vi "recycle_put.vi"(8 "Error In":errorcluster, 9 "Position In":T1) -> (0 "Error Out":errorcluster, 1 "Position out":T1)   [LabVIEW 2019]
uses:
  subVI/move/position cluster.ctl
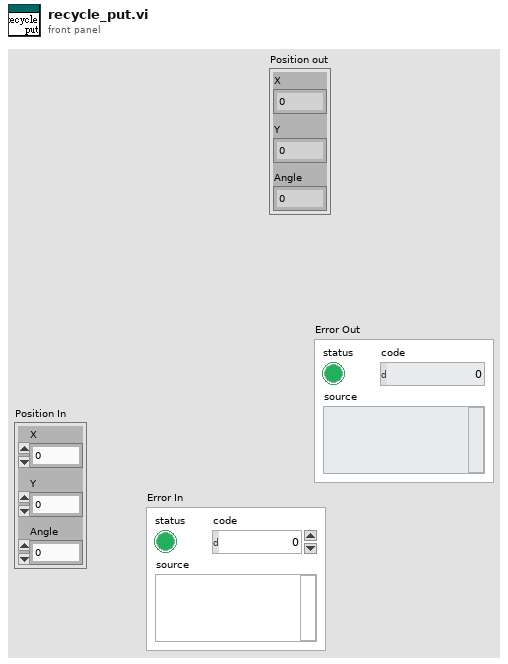
[diagram p1: front panel]
types:
  T1 = typedef "position cluster.ctl" = cluster{"X":dbl, "Y":dbl, "Angle":dbl}
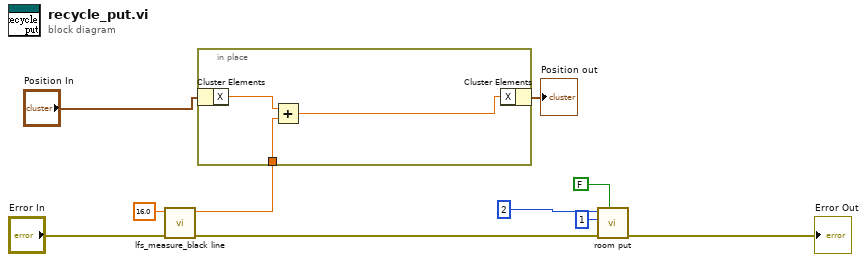
[diagram p0: block diagram]
diagram:
  n1 = call "lfs_measure_black line.vi"("error in (no error)"="Error In", "limit"=16.0) -> ("error out"=w5:errorcluster, "move cm"=w7:dbl)  [unwired: 6 in, 2 out]
  n2 = in-place {
    in-place-border: w7 -> [w12]
    n3 = in-place-cluster #1("Position In") -> ("X"=w13:dbl)
    n4 = Add(x=w13, y=w12) -> (x+y=w11:dbl)
    n5 = in-place-cluster #1("X"=w11) -> (→"Position out":T1)
  }
  n6 = call "room put.vi"("side?"=FALSE, "error in (no error)"=w5, "register address"=1, "put layer"=2) -> ("error out"=→"Error Out":errorcluster)  [unwired: 6 in, 1 out]
